vi "gasoline.vi"() -> ()   [LabVIEW 2021]
panel:
  in  "stop":bool
  in  "установка":T1 {"Стакан" scale=0.0..200.0; "давление газа в сифоне (Па)" scale=0.0..101000.0; "внутренний объем" scale=0.0..300.0}
  out "состояние установки":T2(ring)
  in  "1 копейка":bool
  in  "3 копейки":bool
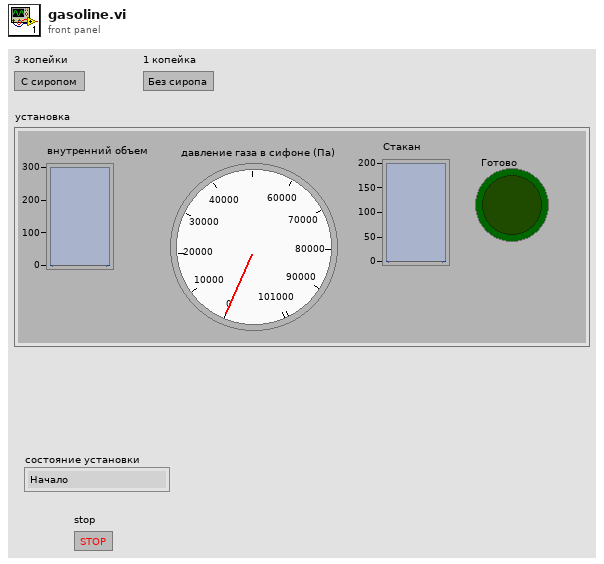
[diagram p1: front panel]
types:
  T1 = cluster{"внутренний объем":dbl, "давление газа в сифоне (Па)":dbl, "Стакан":dbl, "Готово":bool}
  T2 = enum16{"Начало", "заливаем сироп ", "наливаем воду 175", "наливаем воду 200", "газ", "выливаем в стакан", "индикатор", "все"}
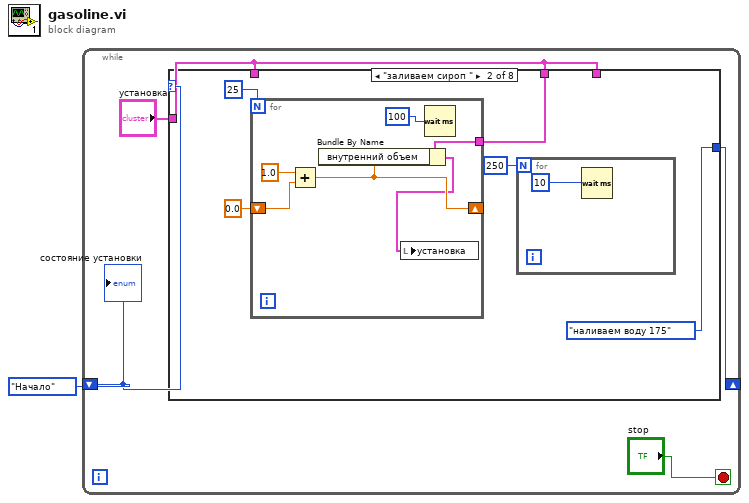
[diagram p0: block diagram]
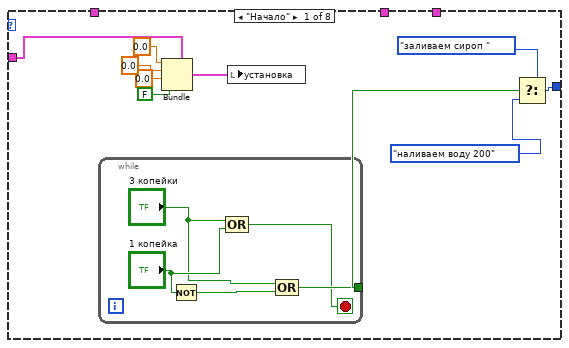
[diagram p2: hidden frame]
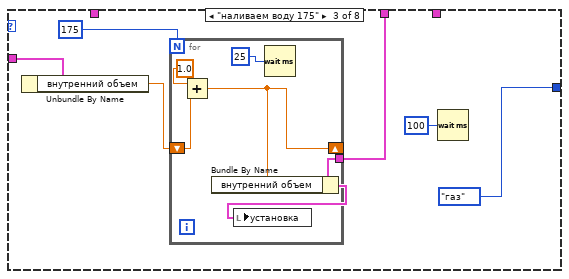
[diagram p3: hidden frame]
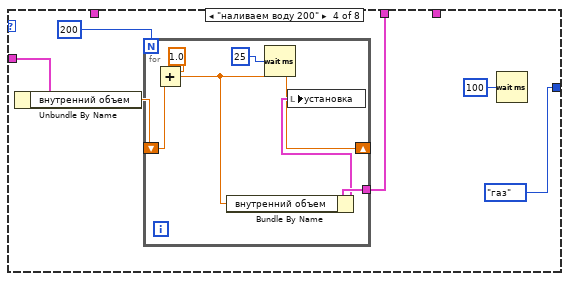
[diagram p4: hidden frame]
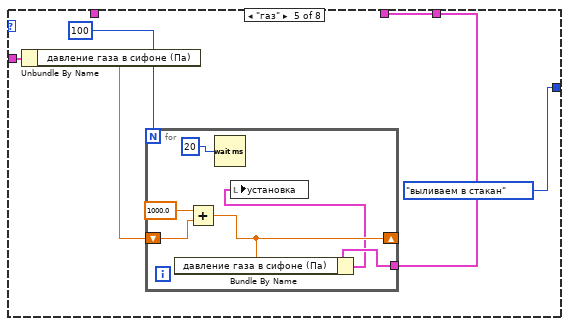
[diagram p5: hidden frame]
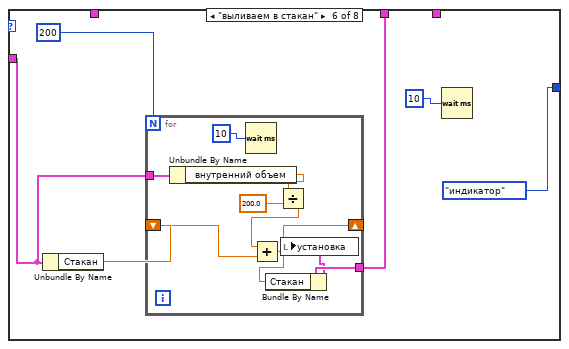
[diagram p6: hidden frame]
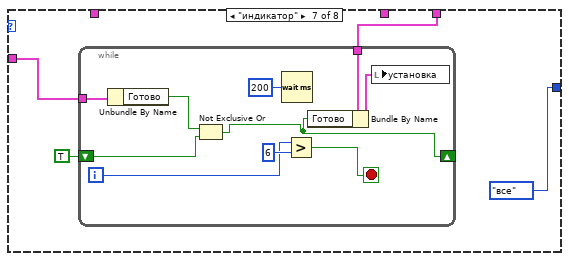
[diagram p7: hidden frame]
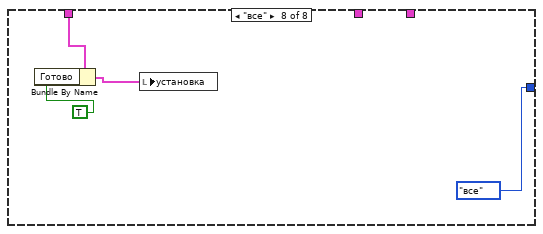
[diagram p8: hidden frame]
diagram:
  n1 = while {
    shift-right: [w4] -> _
    shift-left: T2."Начало" ("состояние установки") -> [w5]
    stop <- "stop" stop-if-true
    n2 = case shown="\"заливаем сироп \"" w5 {
      tunnel: [w12 T2."наливаем воду 175" ("состояние установки") T2."газ" ("состояние установки") T2."газ" ("состояние установки") T2."выливаем в стакан" ("состояние установки") T2."индикатор" ("состояние установки") T2."все" ("состояние установки") T2."все" ("состояние установки")] -> w4
      tunnel: "установка" -> [_ w22 w34 w46 w57 w69 _ _]
      tunnel: "установка" -> [w11 _ w36 w48 w58 w70 w85 _]
      tunnel: "установка" -> [_ _ _ _ _ _ w84 _]
      tunnel: "установка" -> [_ _ _ _ _ _ _ w98]
      frame "Начало" {
        n3 = while {
          tunnel: [w19] -> w15
          stop <- w16 stop-if-true
          n4 = Not(x="1 копейка") -> (.not. x?=w20:bool)
          n5 = Compound Arithmetic op=OR("3 копейки", "1 копейка") -> (w16:bool)
          n6 = Compound Arithmetic op=OR("3 копейки", w20) -> (w19:bool)
        }
        n7 = Bundle(cluster=w11, "внутренний объем"=0.0, "давление газа в сифоне (Па)"=0.0, "Стакан"=0.0, "Готово"=FALSE) -> (w6:T1)
        n8 = local write "установка"(w6) -> ()
        n9 = Select(t=T2."заливаем сироп " ("состояние установки"), s=w15, f=T2."наливаем воду 200" ("состояние установки")) -> (s? t:f=w12:T2)
      }
      frame "заливаем сироп " {
        n10 = for {
          N: 25 -> [_]
          shift-right: [w28] -> _
          shift-left: 0.0 -> [w31]
          tunnel: w22 -> [w29]
          n11 = Add(x=1.0, y=w31) -> (x+y=w28:dbl)
          n12 = Bundle By Name(cluster=w29, "внутренний объем"=w28) -> (w27:T1)
          n13 = local write "установка"(w27) -> ()
          n14 = Wait (ms)(milliseconds to wait=u32 100) -> ()  [unwired: 1 out]
        }
        n15 = for {
          N: 250 -> [_]
          n16 = Wait (ms)(milliseconds to wait=u32 10) -> ()  [unwired: 1 out]
        }
      }
      frame "наливаем воду 175" {
        n17 = Unbundle By Name(w36) -> ("внутренний объем"=w35:dbl)
        n18 = for {
          N: 175 -> [_]
          shift-right: [w40] -> _
          shift-left: w35 -> [w43]
          tunnel: w34 -> [w41]
          n19 = Add(x=1.0, y=w43) -> (x+y=w40:dbl)
          n20 = Bundle By Name(cluster=w41, "внутренний объем"=w40) -> (w39:T1)
          n21 = local write "установка"(w39) -> ()
          n22 = Wait (ms)(milliseconds to wait=u32 25) -> ()  [unwired: 1 out]
        }
        n23 = Wait (ms)(milliseconds to wait=u32 100) -> ()  [unwired: 1 out]
      }
      frame "наливаем воду 200" {
        n24 = Unbundle By Name(w48) -> ("внутренний объем"=w47:dbl)
        n25 = for {
          N: 200 -> [_]
          shift-right: [w51] -> _
          shift-left: w47 -> [w55]
          tunnel: w46 -> [w53]
          n26 = Add(x=1.0, y=w55) -> (x+y=w51:dbl)
          n27 = Bundle By Name(cluster=w53, "внутренний объем"=w51) -> (w52:T1)
          n28 = Wait (ms)(milliseconds to wait=u32 25) -> ()  [unwired: 1 out]
          n29 = local write "установка"(w52) -> ()
        }
        n30 = Wait (ms)(milliseconds to wait=u32 100) -> ()  [unwired: 1 out]
      }
      frame "газ" {
        n31 = Unbundle By Name(w58) -> ("давление газа в сифоне (Па)"=w59:dbl)
        n32 = for {
          N: 100 -> [_]
          shift-right: [w64] -> _
          shift-left: w59 -> [w66]
          tunnel: w57 -> [w63]
          n33 = Add(x=1000.0, y=w66) -> (x+y=w64:dbl)
          n34 = Bundle By Name(cluster=w63, "давление газа в сифоне (Па)"=w64) -> (w62:T1)
          n35 = Wait (ms)(milliseconds to wait=u32 20) -> ()  [unwired: 1 out]
          n36 = local write "установка"(w62) -> ()
        }
      }
      frame "выливаем в стакан" {
        n37 = Unbundle By Name(w70) -> ("Стакан"=w71:dbl)
        n38 = for {
          N: 200 -> [_]
          shift-right: [w75] -> _
          shift-left: w71 -> [w81]
          tunnel: w70 -> [w80]
          tunnel: w69 -> [w76]
          n39 = Unbundle By Name(w80) -> ("внутренний объем"=w79:dbl)
          n40 = Wait (ms)(milliseconds to wait=u32 10) -> ()  [unwired: 1 out]
          n41 = Divide(x=w79, y=200.0) -> (x/y=w77:dbl)
          n42 = Add(x=w77, y=w81) -> (x+y=w75:dbl)
          n43 = Bundle By Name(cluster=w76, "Стакан"=w75) -> (w74:T1)
          n44 = local write "установка"(w74) -> ()
        }
        n45 = Wait (ms)(milliseconds to wait=u32 10) -> ()  [unwired: 1 out]
      }
      frame "индикатор" {
        n46 = while {
          tunnel: w85 -> [w96]
          tunnel: w84 -> [w91]
          shift-right: [w89] -> _
          shift-left: TRUE -> [w87]
          i -> [w92]
          stop <- w93 stop-if-true
          n47 = Unbundle By Name(w96) -> ("Готово"=w88:bool)
          n48 = Not Exclusive Or(1:w87, 2:w88) -> (0:w89:bool)
          n49 = Wait (ms)(milliseconds to wait=u32 200) -> ()  [unwired: 1 out]
          n50 = Greater?(x=w92, y=6) -> (0:w93:bool)
          n51 = Bundle By Name(cluster=w91, "Готово"=w89) -> (w90:T1)
          n52 = local write "установка"(w90) -> ()
        }
      }
      frame "все" {
        n53 = Bundle By Name(cluster=w98, "Готово"=TRUE) -> (w97:T1)
        n54 = local write "установка"(w97) -> ()
      }
    }
    "состояние установки" <- w5
  }
